vi "getID.vi"(8 "error in (no error)":errorcluster, 11 "LLSearch in":refnum<class "LLSearch.lvclass">) -> (0 "error out":errorcluster, 2 "ID":u32, 3 "LLSearch out":refnum<class "LLSearch.lvclass">)   [LabVIEW 2009, in "LLSearch.lvclass"]
uses:
  LLSearch.lvclass
  LLSearch.lvclass/LLSearch.ctl
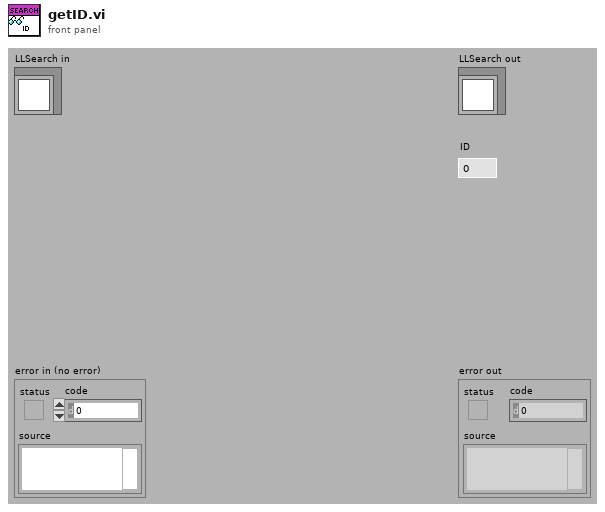
[diagram p1: front panel]
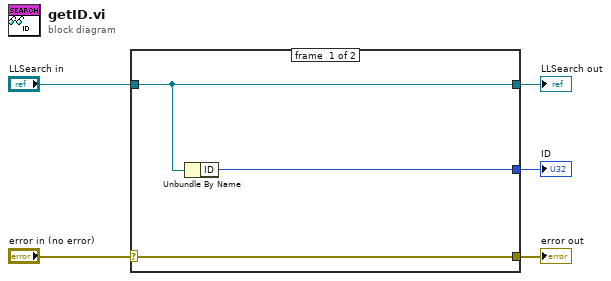
[diagram p0: block diagram]
diagram:
  n1 = case shown="No Error" "error in (no error)" {
    selector: "error in (no error)" -> [w8 w9]
    tunnel: [w8 w9] -> w4
    tunnel: [w7 w10] -> w2
    tunnel: "LLSearch in" -> [w7 w10]
    tunnel: [w6 _] -> w1
    frame #0 {
      n2 = Unbundle By Name(w7) -> ("ID"=w6:u32)
    }
    frame #1 {
    }
  }
  "error out" <- w4
  "LLSearch out" <- w2
  "ID" <- w1
